vi "subStepper Motor Init.vi"(8 "error in":errorcluster, 10 "Numeric":dbl, 11 "Arduino Resource":T1={"VISA resource"="", "Board Type"=enum."Uno", "Connection Type"=enum."USB / Serial", "Bytes Per Packet (15)"=15}) -> (0 "error out":errorcluster, 3 "Arduino Resource 2":T1={"VISA resource"="", "Board Type"=enum."Uno", "Connection Type"=enum."USB / Serial", "Bytes Per Packet (15)"=15})   [LabVIEW 2016]
uses:
  <vilib>/LabVIEW Interface for Arduino/Type Defs/Arduino Resource.ctl
  <vilib>/LabVIEW Interface for Arduino/Type Defs/Board Type.ctl
  <vilib>/LabVIEW Interface for Arduino/LabVIEW Interface for Arduino.lvlib
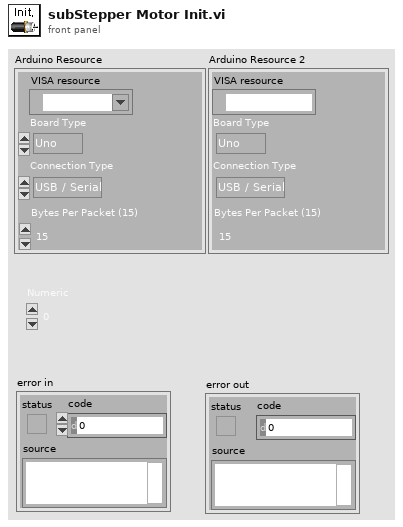
[diagram p1: front panel]
types:
  T1 = typedef "LabVIEW Interface for Arduino.lvlib/Arduino Resource.ctl" = cluster{"VISA resource":refnum<visa-resource-name>, "Board Type":T2, "Connection Type":enum8{"USB / Serial"}, "Bytes Per Packet (15)":u8}
  T2 = typedef "LabVIEW Interface for Arduino.lvlib/Board Type.ctl" = enum16{"Uno", "Dimuelanove w/Atmega 328", "Mega 2560"}
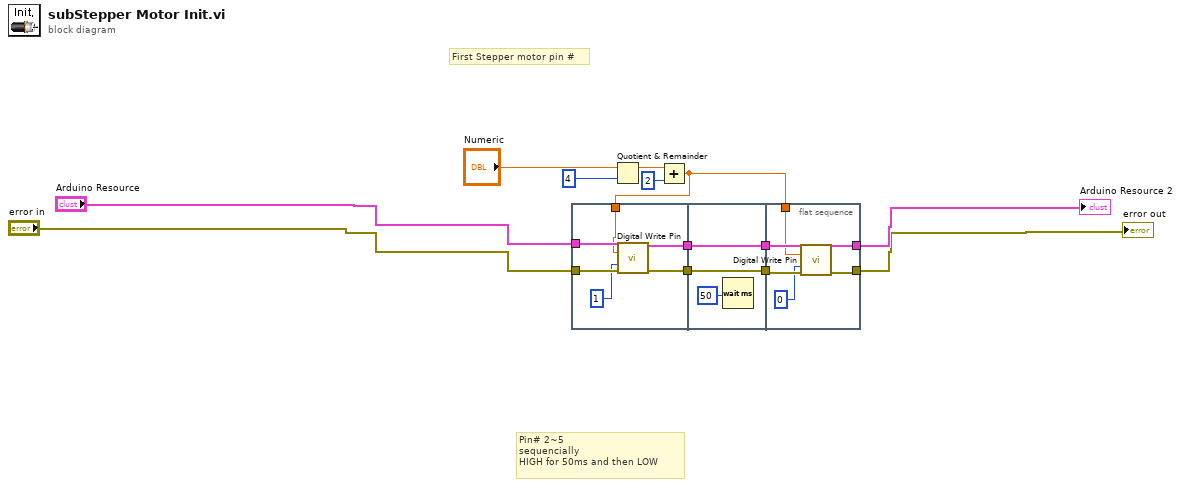
[diagram p0: block diagram]
diagram:
  # "Pin# 2~5\nsequencially\nHIGH for 50ms and then LOW"
  # "First Stepper motor pin #"
  n1 = flat-sequence {
    tunnel: "Arduino Resource" -> [w19]
    tunnel: "error in" -> [w18]
    tunnel: [w17] -> w9
    tunnel: [w16] -> w8
    tunnel: w2 -> [w15]
    tunnel: w9 -> [w22]
    tunnel: w8 -> [w21]
    tunnel: [w22] -> w7
    tunnel: [w21] -> w6
    tunnel: [w26] -> w12
    tunnel: [w27] -> w13
    tunnel: w7 -> [w28]
    tunnel: w6 -> [w25]
    tunnel: w2 -> [w24]
    frame #0 {
      n2 = call <vilib>:"Digital Write Pin.vi"("Arduino Resource"=w19, "Digital I/O Pin (0)"=w15, "Value (0)"=1, "error in"=w18) -> ("Arduino Resource"=w17:T1, "error out"=w16:errorcluster)  [unwired: 10 in]
    }
    frame #1 {
      n3 = Wait (ms)(milliseconds to wait=50) -> ()  [unwired: 1 out]
    }
    frame #2 {
      n4 = call <vilib>:"Digital Write Pin.vi"("Arduino Resource"=w28, "Digital I/O Pin (0)"=w24, "Value (0)"=0, "error in"=w25) -> ("Arduino Resource"=w27:T1, "error out"=w26:errorcluster)  [unwired: 10 in]
    }
  }
  n5 = Quotient & Remainder(x="Numeric", y=4) -> (x-y*floor(x/y)=w4:dbl)  [unwired: 1 out]
  n6 = Add(x=w4, y=2) -> (x+y=w2:dbl)
  "Arduino Resource 2" <- w13
  "error out" <- w12
